vi "buildPathFromStrArr.vi"(9 "String Array":string[](array[string]), 11 "Root Path":path) -> (3 "Absolute Path":path)   [LabVIEW 2018]
doc: "Build the absolute path from the root and following string array."
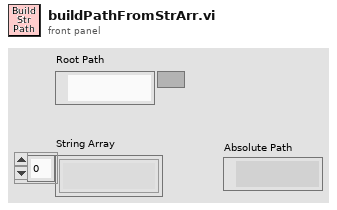
[diagram p1: front panel]
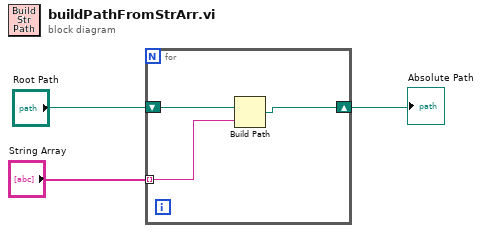
[diagram p0: block diagram]
diagram:
  n1 = for {
    shift-right: [w4] -> w1
    shift-left: "Root Path" -> [w6]
    tunnel: "String Array" -> [w5] mode=indexing
    n2 = Build Path(base path=w6, name or relative path=w5) -> (appended path=w4:path)
  }
  "Absolute Path" <- w1
